vi "SHUmrechnen-11-15.vi"(6 "TemperaturSH[°C]":dbl, 7 "SpannungSH[V]":dbl, 9 "Koeff2":dbl, 10 "Koeff1":dbl, 11 "Koeff0":dbl) -> (1 "SpannungSH[V]":fxp<+/-,16,4> format="%.14g", 3 "TemperaturSH[°C]":dbl)   [LabVIEW 2010]
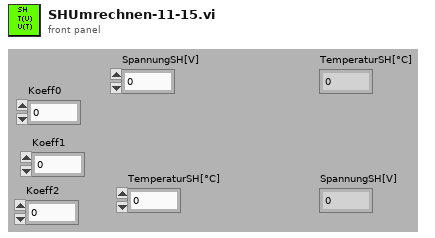
[diagram p1: front panel]
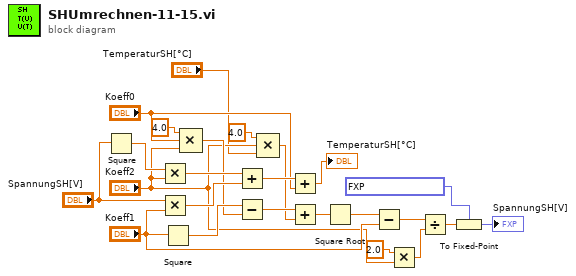
[diagram p0: block diagram]
diagram:
  n1 = Square(x="SpannungSH[V]") -> (x^2=w21:dbl)
  n2 = Multiply(x=w21, y="Koeff2") -> (x*y=w22:dbl)
  n3 = Multiply(x="SpannungSH[V]", y="Koeff1") -> (x*y=w23:dbl)
  n4 = Square(x="Koeff1") -> (x^2=w18:dbl)
  n5 = Compound Arithmetic op=MULTIPLY(4.0, "Koeff0", "Koeff2") -> (w17:dbl)
  n6 = Add(x=w22, y=w23) -> (x+y=w24:dbl)
  n7 = Subtract(x=w18, y=w17) -> (x-y=w16:dbl)
  n8 = Compound Arithmetic op=MULTIPLY(4.0, "Koeff2", "TemperaturSH[°C]") -> (w15:dbl)
  n9 = Add(x=w24, y="Koeff0") -> (x+y=→"TemperaturSH[°C]":dbl)
  n10 = Add(x=w16, y=w15) -> (x+y=w14:dbl)
  n11 = Square Root(x=w14) -> (sqrt(x)=w13:dbl)
  n12 = Subtract(x=w13, y="Koeff1") -> (x-y=w12:dbl)
  n13 = Multiply(x=2.0, y="Koeff2") -> (x*y=w10:dbl)
  n14 = Divide(x=w12, y=w10) -> (x/y=w9:dbl)
  n15 = To Fixed-Point(fixed-point type=fxp<+/-,16,4> 0.0 ("USetp [V]Mach1"), number=w9) -> (fixed-point=→"SpannungSH[V]":fxp<+/-,16,4>)
